vi "图像属性操作.vi"() -> ()   [LabVIEW 2018]
uses:
  <vilib>/vision/NI_Vision_Development_Module.lvlib
panel:
  out "error out":errorcluster
  in  "error in (no error)":errorcluster
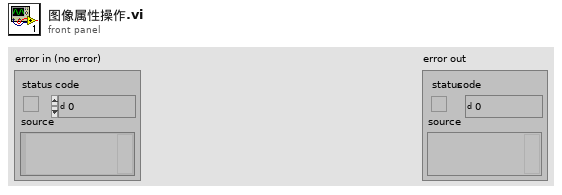
[diagram p1: front panel]
types:
  T1 = typedef "Image Type" = u32
  T2 = typedef "IMAQ Image.ctl" = refnum<image>
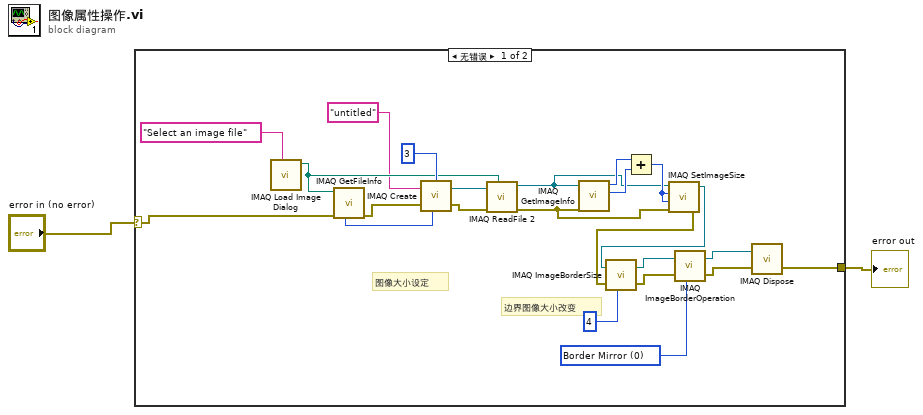
[diagram p0: block diagram]
diagram:
  n1 = case shown="无错误" "error in (no error)" {
    selector: "error in (no error)" -> [w21 w26]
    tunnel: [w6 w26] -> w1
    frame No Error {
      w8 = u32 0 items=["Border Mirror", "Border Copy", "Border Clear"] ("Function")
      # "边界图像大小改变"
      # "图像大小设定"
      n2 = call "IMAQ Load Image Dialog"("Prompt"="Select an image file") -> ("Path"=w4:path)  [unwired: 8 in, 2 out]
      n3 = call "IMAQ GetFileInfo"("error in (no error)"=w21, "File Path"=w4) -> ("error out"=w24:errorcluster, "Image Type"=w23:T1)  [unwired: 3 in, 5 out]
      n4 = call "IMAQ Create"("Border Size"=3, "Image Name"="untitled", "Image Type"=w23, "error in (no error)"=w24) -> ("New Image"=w17:T2, "error out"=w16:errorcluster)  [unwired: 1 in]
      n5 = call "IMAQ ReadFile 2"("File Path"=w4, "error in (no error)"=w16, "Image"=w17) -> ("error out"=w14:errorcluster, "Image Out"=w15:T2)  [unwired: 4 in, 3 out]
      n6 = call "IMAQ GetImageInfo"("error in (no error)"=w14, "Image"=w15) -> ("Y Resolution"=w19:i32, "X Resolution"=w20:i32)  [unwired: 2 in, 6 out]
      n7 = Add(x=w20, y=w19) -> (x+y=w18:i32)
      n8 = call "IMAQ SetImageSize"("error in (no error)"=w14, "Y Resolution"=w18, "X Resolution"=w18, "Image"=w15) -> ("error out"=w12:errorcluster, "Image Out"=w13:T2)  [unwired: 1 in]
      n9 = call "IMAQ ImageBorderSize"("Image"=w13, "Image border size in"=4, "error in (no error)"=w12) -> ("Image Out"=w11:T2, "error out"=w10:errorcluster)  [unwired: 1 in, 1 out]
      n10 = call "IMAQ ImageBorderOperation"("Image"=w11, "Function"=w8, "error in (no error)"=w10) -> ("Image Out"=w9:T2, "error out"=w7:errorcluster)  [unwired: 2 in]
      n11 = call "IMAQ Dispose"("Image"=w9, "error in (no error)"=w7) -> ("error out"=w6:errorcluster)  [unwired: 4 in]
    }
    frame Error {
    }
  }
  "error out" <- w1
